vi "Memory.vi"(7 "Action (get)":enum8{"get", "set"}(ring), 8 "error in (no error)":errorcluster, 11 "skvc in":string[][](array[string])) -> (0 "error out":errorcluster, 3 "skvc out":string[][](array[string]))   [LabVIEW 2021, in "Config.lvlib"]
uses:
  Config.lvlib
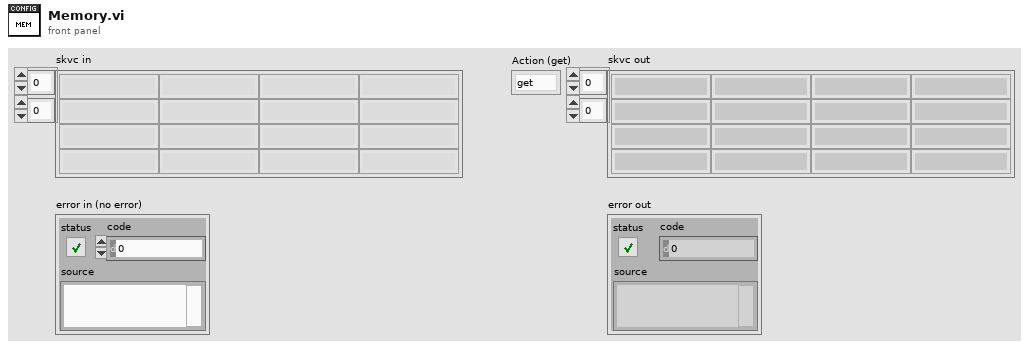
[diagram p1: front panel]
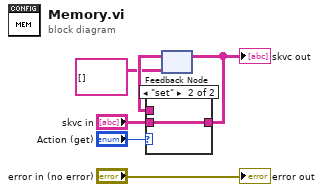
[diagram p0: block diagram]
diagram:
  n1 = feedback #1(string[][] [] ("skvc")) -> (w4:string[][])
  n2 = case shown="\"set\"" "Action (get)" {
    tunnel: [w7 w8] -> w3
    tunnel: "skvc in" -> [_ w8]
    tunnel: w4 -> [w7 _]
    frame "get" {
    }
    frame "set" {
    }
  }
  "skvc out" <- w3
  n3 = feedback-in #1(w3) -> ()
  "error out" <- "error in (no error)"
